vi "NanonisProperties_rawspeed.vi"(0 "Application ref in":refnum<vi>, 5 "Position (nm)":cluster{"X":dbl, "Z":dbl, "Y":dbl}, 11 "error in (no error)":errorcluster, 12 "Z Write?":bool) -> (4 "Application ref out":refnum<vi>, 15 "error out":errorcluster)   [LabVIEW 2017]
uses:
  <userlib>/Nanonis Prog Interface V5/Nanonis Prog Interface.lvlib
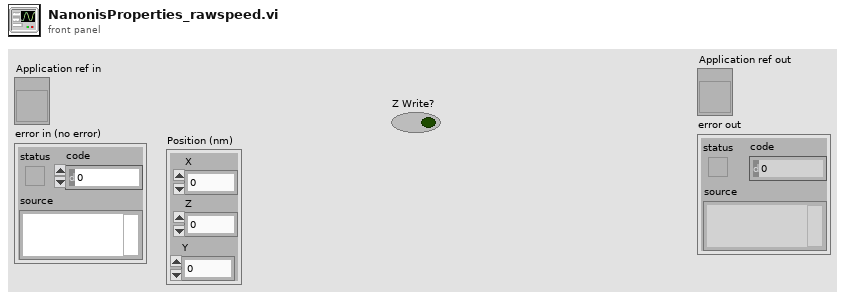
[diagram p1: front panel]
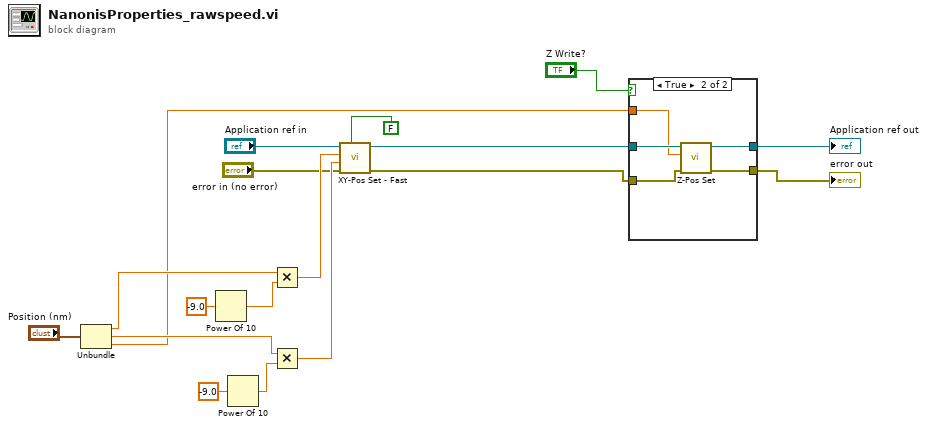
[diagram p0: block diagram]
diagram:
  n1 = Unbundle("Position (nm)") -> ("X"=w7:dbl, "Z"=w6:dbl, "Y"=w5:dbl)
  n2 = Power Of 10(x=-9.0) -> (10^x=w17:dbl)
  n3 = Power Of 10(x=-9.0) -> (10^x=w15:dbl)
  n4 = Multiply(x=w7, y=w17) -> (x*y=w13:dbl)
  n5 = Multiply(x=w6, y=w15) -> (x*y=w12:dbl)
  n6 = call <userlib>:"XY-Pos Set - Fast.vi"("Wait end-of-motion (T=True)"=FALSE, "error in (no error)"="error in (no error)", "Y (m)"=w12, "X (m)"=w13, "Application ref in"="Application ref in") -> ("error out"=w1:errorcluster, "Application ref out"=w2:refnum<vi>)  [unwired: 4 in]
  n7 = case shown="True" "Z Write?" {
    tunnel: w2 -> [w20 w25]
    tunnel: [w20 w24] -> w11
    tunnel: [w19 w23] -> w10
    tunnel: w5 -> [_ w22]
    tunnel: w1 -> [w19 w21]
    frame False {
    }
    frame True {
      n8 = call <userlib>:"Z-Pos Set.vi"("error in (no error)"=w21, "Z position (m)"=w22, "Application ref in"=w25) -> ("error out"=w23:errorcluster, "Application ref out"=w24:refnum<vi>)  [unwired: 7 in]
    }
  }
  "Application ref out" <- w11
  "error out" <- w10
